vi "EncoderRefNum_Simulation_Global.vi"(0 "menu":enum16{"set", "get", "delete"}(ring)=enum."get", 5 "Encoder":T1, 7 "Rate in":dbl, 9 "Maxon Encoder Set":refnum<class "Maxon Encoder.lvclass">, 11 "error in (no error)":errorcluster) -> (8 "Rate out":dbl, 10 "Maxon Encoder Get":refnum<class "Maxon Encoder.lvclass">, 15 "error out":errorcluster)   [LabVIEW 2017]
doc: "Sets a reference into a registry, gets a reference from a registry, or deletes a reference from a registry. The reference is accessed by name, and can be given any unique name.\n\nThis software is licensed. Open the labview\\readme\\WPI Robotics Library Open Source License.txt file for more information."
uses:
  <instrlib>/Maxon Encoder/HAIOL/Maxon Encoder.lvclass
  <vilib>/Rock Robotics/SystemInterfaces/Encoder/FPGA_EncoderIdx.ctl
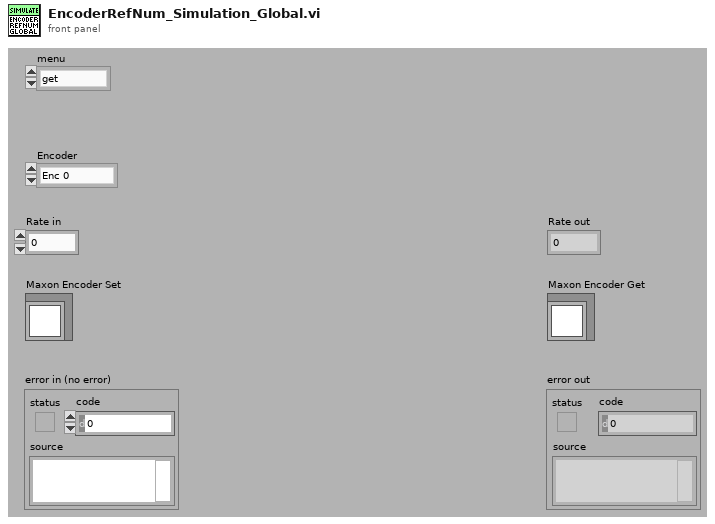
[diagram p1: front panel]
types:
  T1 = typedef "FPGA_EncoderIdx.ctl" = enum8{"Enc 0", "Enc 1", "Enc 2", "Enc 3", "Enc 4", "Enc 5", "Enc 6", "Enc 7", "Invalid"}
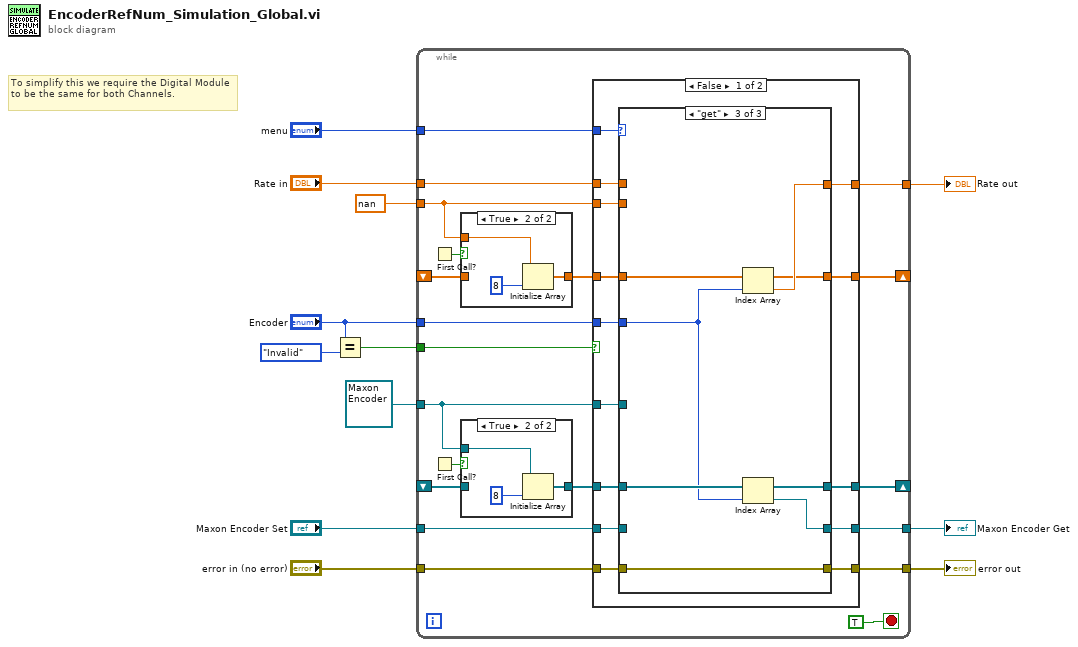
[diagram p0: block diagram]
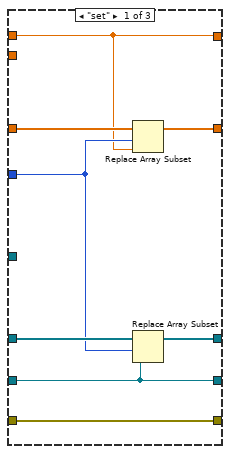
[diagram p3: hidden frame]
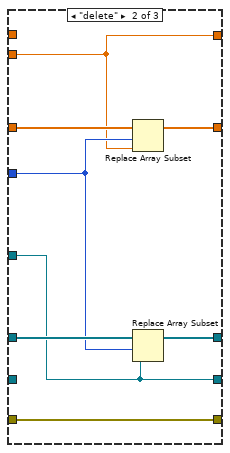
[diagram p4: hidden frame]
diagram:
  # "To simplify this we require the Digital Module to be the same for both Channels."
  n1 = Equal?(x="Encoder", y=FPGA_EncoderIdx."Invalid" ("Encoder")) -> (x = y?=w4:bool)
  n2 = while {
    tunnel: "Maxon Encoder Set" -> [w32]
    tunnel: "error in (no error)" -> [w28]
    shift-right: [w31] -> _
    shift-left: _ -> [w23]
    tunnel: [w30] -> w7
    tunnel: "menu" -> [w29]
    tunnel: [w27] -> w11
    tunnel: "Encoder" -> [w22]
    tunnel: w4 -> [w21]
    tunnel: refnum<class "Maxon Encoder.lvclass"> refnum ("Maxon Encoder out") -> [w20]
    tunnel: [w17] -> w3
    tunnel: "Rate in" -> [w16]
    shift-right: [w15] -> _
    shift-left: _ -> [w14]
    tunnel: nan ("Rate in") -> [w13]
    stop <- TRUE stop-if-true
    n3 = First Call?() -> (First Call?: T/F=w19:bool)
    n4 = First Call?() -> (First Call?: T/F=w25:bool)
    n5 = case shown="True" w19 {
      tunnel: [w33 w35] -> w18
      tunnel: w14 -> [w33 _]
      tunnel: w13 -> [_ w34]
      frame False {
      }
      frame True {
        n6 = Initialize Array(w34, 8 ("dimension size")) -> (w35:dbl[])
      }
    }
    n7 = case shown="True" w25 {
      tunnel: [w78 w80] -> w24
      tunnel: w23 -> [w78 _]
      tunnel: w20 -> [_ w79]
      frame False {
      }
      frame True {
        n8 = Initialize Array(w79, 8 ("dimension size")) -> (w80:refnum<class "Maxon Encoder.lvclass">[])
      }
    }
    n9 = case shown="False" w21 {
      tunnel: w32 -> [w50 _]
      tunnel: [w49 w77] -> w31
      tunnel: [w48 w75] -> w30
      tunnel: w29 -> [w47 _]
      tunnel: w28 -> [w46 w76]
      tunnel: [w45 w76] -> w27
      tunnel: w24 -> [w44 w77]
      tunnel: w22 -> [w43 _]
      tunnel: w20 -> [w42 w75]
      tunnel: w18 -> [w41 w74]
      tunnel: [w40 w73] -> w17
      tunnel: w16 -> [w39 _]
      tunnel: [w38 w74] -> w15
      tunnel: w13 -> [w37 w73]
      frame False {
        n10 = case shown="\"get\"" w47 {
          tunnel: w50 -> [w56 _ _]
          tunnel: [w57 w65 w72] -> w49
          tunnel: w44 -> [w58 w66 w72]
          tunnel: [w56 w63 w71] -> w48
          tunnel: [w55 w64 w70] -> w45
          tunnel: w46 -> [w55 w64 w70]
          tunnel: w43 -> [w53 w60 w69]
          tunnel: w42 -> [_ w63 _]
          tunnel: w41 -> [w54 w62 w67]
          tunnel: [w51 w59 w68] -> w40
          tunnel: w39 -> [w51 _ _]
          tunnel: [w52 w61 w67] -> w38
          tunnel: w37 -> [_ w59 _]
          frame "set" {
            n11 = Replace Array Subset(array=w54, new element=w51, index=w53) -> (w52:dbl[])
            n12 = Replace Array Subset(array=w58, new element=w56, index=w53) -> (w57:refnum<class "Maxon Encoder.lvclass">[])
          }
          frame "delete" {
            n13 = Replace Array Subset(array=w62, new element=w59, index=w60) -> (w61:dbl[])
            n14 = Replace Array Subset(array=w66, new element=w63, index=w60) -> (w65:refnum<class "Maxon Encoder.lvclass">[])
          }
          frame "get" {
            n15 = Index Array(array=w67, index=w69) -> (element=w68:dbl)
            n16 = Index Array(array=w72, index=w69) -> (element=w71:refnum<class "Maxon Encoder.lvclass">)
          }
        }
      }
      frame True {
        # "Do nothing if different modules."
        # "Do nothing if channel is Invalid."
      }
    }
  }
  "error out" <- w11
  "Maxon Encoder Get" <- w7
  "Rate out" <- w3
